vi "RescaleSpectrometerGraphX.vi"(11 "Spectrometer wavelengths":sgl[][](array[numeric])) -> (2 "Numeric 2":sgl, 3 "Numeric":sgl)   [LabVIEW 2012]
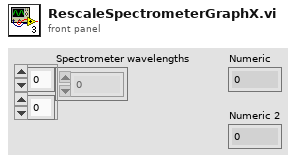
[diagram p1: front panel]
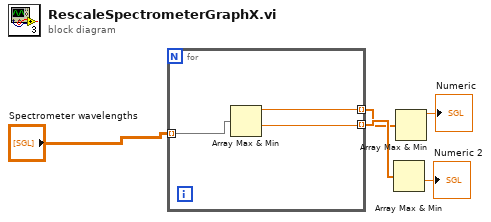
[diagram p0: block diagram]
diagram:
  n1 = for {
    tunnel: "Spectrometer wavelengths" -> [w8] mode=indexing
    tunnel: [w7] -> w2 mode=indexing
    tunnel: [w6] -> w3 mode=indexing
    n2 = Array Max & Min(array=w8) -> (max value=w7:sgl, min value=w6:sgl)  [unwired: 2 out]
  }
  n3 = Array Max & Min(array=w3) -> (min value=→"Numeric 2":sgl)  [unwired: 3 out]
  n4 = Array Max & Min(array=w2) -> (max value=→"Numeric":sgl)  [unwired: 3 out]
